vi "multi2.vi"() -> ()   [LabVIEW 2020]
uses:
  <vilib>/rvi/IPIntegrationNode/IPINode_Typedef/niFpgaIPINodeSupportedFamilies.ctl
  <vilib>/rvi/Emulation/niFpgaGetClockAttributes.vi
  <vilib>/rvi/Emulation/niFpgaSctlEmulationGetInTimedLoop.vi
  <vilib>/rvi/Emulation/niFpgaEmulationReportErrorSimple.vi
  <vilib>/rvi/IPIntegrationNode/IPINode_Utilities/niFpgaIPINodeSimCore.vi
  <vilib>/rvi/Emulation/niFpgaCriticalErrorInLSC.vi
  <vilib>/rvi/IPIntegrationNode/IPINode_Xnode/niFpgaIPINode.xnode
  MULTIPLY/MULTIPLY.srcs/sources_1/new/multiply_27SimFiles/xsim.dir/multiwrapper/xsimk5616B772008E4FE895D1368191252568.dll
  <vilib>/rvi/Analysis/measure/butterworth/XNode/niFpgaButterworthFilter.xnode
panel:
  out "appended array 2":cluster{sgl, sgl}(graph)={-113261490.0, -277554500.0} caption="appended array"
  out "appended array":cluster{sgl, sgl}(graph)={-30852.0, 5007.0}
  in  "frequency(kHz) 2":fxp<+,32,16>=90.0
  in  "frequency(kHz)":fxp<+,32,16>=100.0
  in  "stop":bool
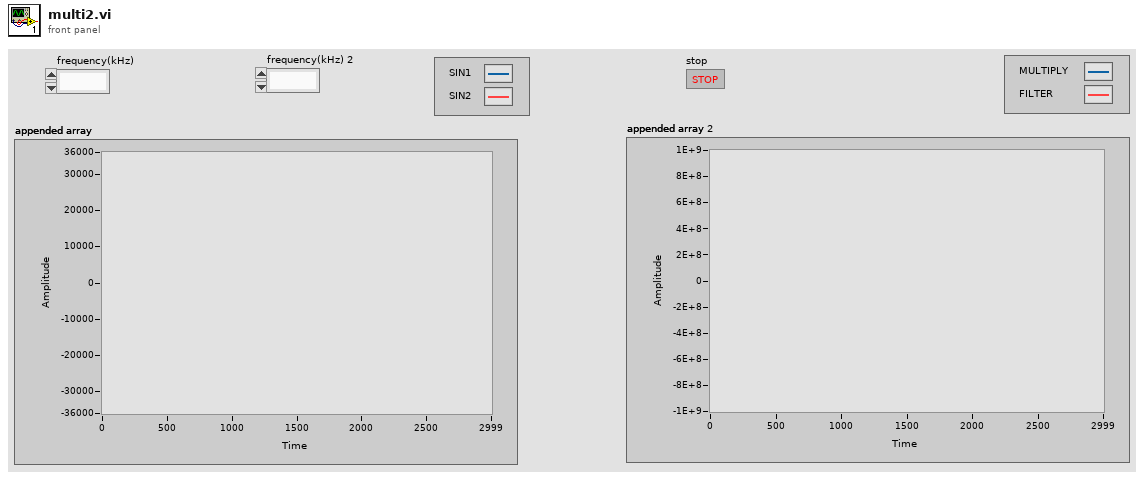
[diagram p1: front panel]
types:
  T1 = typedef "niFpgaIPINodeSupportedFamilies.ctl" = cluster{"unlimited?":bool, "supported targets":string[]}
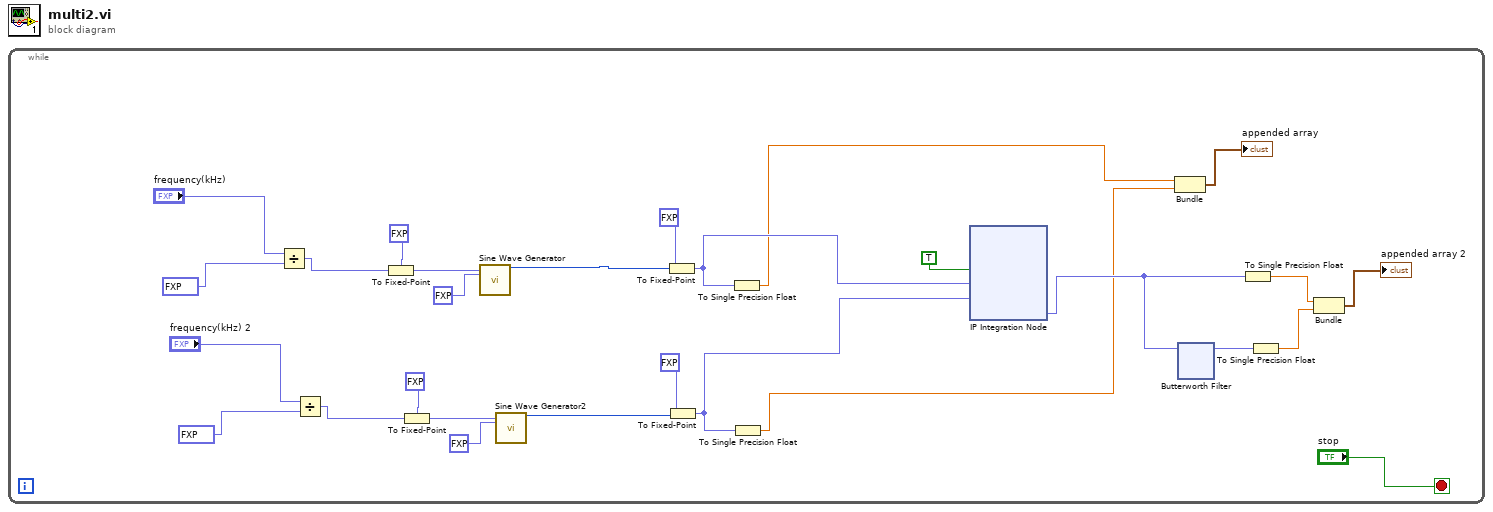
[diagram p0: block diagram]
diagram:
  n1 = while {
    stop <- "stop" stop-if-true
    n2 = Divide(x="frequency(kHz)", y=fxp<+,32,16> 40000.0 ("frequency (periods/tick)")) -> (x/y=w20:fxp<+,64,32>)
    n3 = Divide(x="frequency(kHz) 2", y=fxp<+,32,16> 40000.0 ("frequency (periods/tick)")) -> (x/y=w8:fxp<+,64,32>)
    n4 = To Fixed-Point(fixed-point type=fxp<+,32,0> 0.0 ("frequency (periods/tick)"), number=w20) -> (fixed-point=w18:fxp<+,32,0>)
    n5 = To Fixed-Point(fixed-point type=fxp<+,32,0> 0.0 ("frequency (periods/tick)"), number=w8) -> (fixed-point=w10:fxp<+,32,0>)
    n6 = call "Sine Wave Generator"("frequency (periods/tick)"=w18, "phase offset (periods)"=fxp<+,32,0> 0.0) -> ("sine out"=w14:i16)  [unwired: 13 in]
    n7 = call "Sine Wave Generator2"("frequency (periods/tick)"=w10, "phase offset (periods)"=fxp<+,32,0> 0.0) -> ("sine out"=w7:i16)  [unwired: 13 in]
    n8 = To Fixed-Point(fixed-point type=fxp<+/-,16,16> 0.0, number=w14) -> (fixed-point=w25:fxp<+/-,16,16>)
    n9 = To Fixed-Point(fixed-point type=fxp<+/-,16,16> 0.0, number=w7) -> (fixed-point=w23:fxp<+/-,16,16>)
    n10 = To Single Precision Float(number=w25) -> (single precision float=w6:sgl)
    n11 = To Single Precision Float(number=w23) -> (single precision float=w5:sgl)
    n12 = xnode "IP Integration Node"("cEn"=TRUE, "sig_i_1"=w25, "sig_i_2"=w23) -> ("sig_o"=w22:fxp<+/-,32,32>)
    n13 = Bundle(w6, w5) -> (→"appended array":cluster{sgl, sgl})  [unwired: 1 in]
    n14 = xnode "Butterworth Filter"("input data"=w22) -> ("output data"=w21:fxp<+/-,32,32>)  [unwired: 2 in]
    n15 = To Single Precision Float(number=w22) -> (single precision float=w2:sgl)
    n16 = To Single Precision Float(number=w21) -> (single precision float=w1:sgl)
    n17 = Bundle(w2, w1) -> (→"appended array 2":cluster{sgl, sgl})  [unwired: 1 in]
  }
